vi "Parse pyWebscraper data.vi"(6 "Row Type":T1, 7 "Column Type":T2, 8 "error in (no error)":errorcluster, 10 "2D Array":string[][](array[string])) -> (0 "error out":errorcluster, 2 "element":string)   [LabVIEW 2016, in "Webscraper.lvlib"]
uses:
  Webscraper.lvlib
  Type Definitions/Column Type.ctl
  Type Definitions/Row Type.ctl
  <vilib>/Utility/error.llb/Error Cluster From Error Code.vi
  <vilib>/ErrorRing/Error Ring.xnode
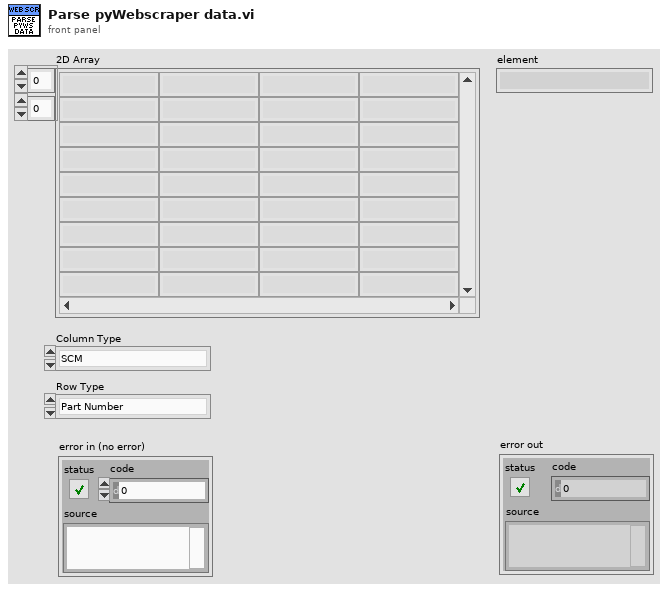
[diagram p1: front panel]
types:
  T1 = typedef "Webscraper.lvlib/Row Type.ctl" = enum16{"Part Number", "Serial Number", "Manufacturing Info", "Manufacturer Name", "Model Revision", "Primary Revision", "Secondary Revision", "LED Status", "Operation", "Current Turn On Time", "Total Turn On Time", "Temperature", "Output Voltage", "Output Current", "Input Voltage", "Input Voltage Type", "Input Power applied", "DC Output ON Cycles", "Output Short Circuit Protection", "Output Over Voltage Protection", "Power Boost", "Over-Temperature Protection", "PS#1 Current High", "PS#1 Temperature High", "PS#1 Input Voltage High", "PS#1 Input Voltage Low", "PS#1 Current Change Threshold", "PS#1 Alarm Enable/Disable", "PS#2 Current High", "PS#2 Temperature High", "PS#2 Input Voltage High", "PS#2 Input Voltage Low", "PS#2 Current Change Threshold", "PS#2 Alarm Enable/Disable", "SCM Temperature High", "SCM Average Temperature Limit", "SCM Alarm Enable/Disable", "Redundancy Alarm Enable/Disable"}
  T2 = typedef "Column Type.ctl" = enum16{"SCM", "PS#1", "PS#2", "Name", "Threshold/Status", "Value", "Unit"}
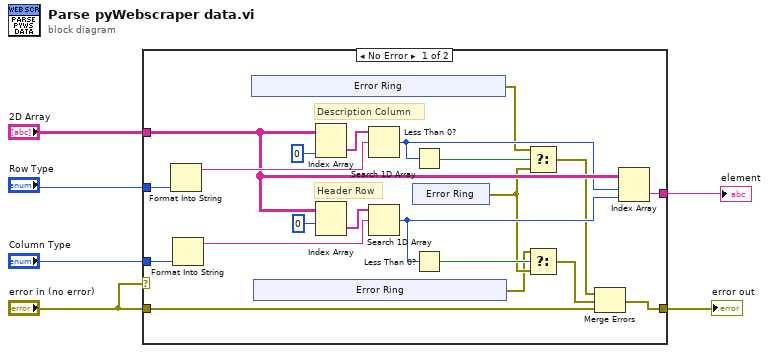
[diagram p0: block diagram]
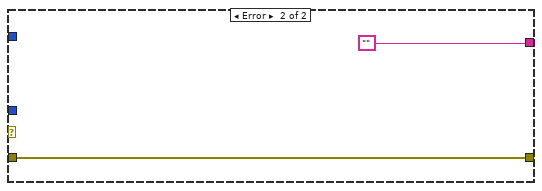
[diagram p2: hidden frame]
diagram:
  n1 = case shown="No Error" "error in (no error)" {
    tunnel: "error in (no error)" -> [w8 w40]
    tunnel: [w7 w40] -> w6
    tunnel: "Row Type" -> [w26 _]
    tunnel: "Column Type" -> [w24 _]
    tunnel: "2D Array" -> [w18 _]
    tunnel: [w19 ""] -> w3
    frame No Error {
      # "Description Column"
      # "Header Row"
      n2 = Format Into String(w26) -> (resulting string=w21:string)  [unwired: 3 in, 1 out]
      n3 = Format Into String(w24) -> (resulting string=w20:string)  [unwired: 3 in, 1 out]
      n4 = xnode "Error Ring"() -> ("error out"=w14:errorcluster)
      n5 = xnode "Error Ring"() -> ("error out"=w11:errorcluster)
      n6 = Index Array(array=w18, index (col)=0 ("disabled index (col)")) -> (element=w22:string[])  [unwired: 1 in]
      n7 = Index Array(array=w18, index (row)=0) -> (element=w23:string[])  [unwired: 1 in]
      n8 = Search 1D Array(1D array=w22, element=w21) -> (index of element=w16:i32)  [unwired: 1 in]
      n9 = Search 1D Array(1D array=w23, element=w20) -> (index of element=w17:i32)  [unwired: 1 in]
      n10 = xnode "Error Ring"() -> ("error out"=w12:errorcluster)
      n11 = Less Than 0?(x=w16) -> (x < 0?=w15:bool)
      n12 = Less Than 0?(x=w17) -> (x < 0?=w13:bool)
      n13 = Select(t=w14, s=w15, f=w12) -> (s? t:f=w10:errorcluster)
      n14 = Select(t=w11, s=w13, f=w12) -> (s? t:f=w9:errorcluster)
      n15 = Merge Errors(w10, w9, w8) -> (w7:errorcluster)
      n16 = Index Array(array=w18, index (row)=w16, index (col)=w17) -> (element=w19:string)
    }
    frame Error {
    }
  }
  "error out" <- w6
  "element" <- w3
